vi "LDA_Angle_Checks.vi"(0 "Vg1":dbl[](array[numeric])=[-0.9913846154927373, -0.08722653267640797, -0.09771425771896834] format="%#.3g", 1 "Vg2":dbl[](array[numeric])=[-0.987756229722306, 0.06610682889995216, -0.1413064677131501] format="%#.3g", 2 "Vb1":dbl[](array[numeric])=[-0.9989930425665134, 0.011295311772511737, -0.04342023532481111] format="%#.3g", 3 "Vb2":dbl[](array[numeric])=[-0.9801478026485297, -0.032415015548967537, -0.19560049010730732] format="%#.3g") -> (6 "Vp from Greens":dbl[](array[numeric])=[-0.9927304194336236, -0.01059357268028935, -0.11989199535001964] format="%.3f", 7 "Vp from Blues":dbl[](array[numeric])=[-0.9927304194336236, -0.010593572680289348, -0.11989199535001965] format="%.3f", 8 "Angle between beam planes (deg)":dbl=90.0 format="%#.3g", 9 "Vp difference (G-B)":dbl[](array[numeric])=[0.0, -1.734723475976807e-18, 1.3877787807814457e-17] format="%_3f", 10 "Angle of spot B1 corner (deg)":dbl=89.99999914622636 format="%#.3g", 11 "Angle of spot B2 corner (deg)":dbl=90.0 format="%#.3g", 12 "Angle of spot G1 corner (deg)":dbl=90.0 format="%#.3g", 13 "Angle of spot G2 corner (deg)":dbl=89.99999914622636 format="%#.3g", 14 "Green divergence angle (deg)":dbl=9.14556525944418 format="%#.3g", 15 "Blue divergence angle (deg)":dbl=9.14556525944422 format="%#.3g", 16 "Angle between Vg1 and Vb1 (deg)":dbl=6.4634547293452185 format="%#.3g", 17 "Angle between Vg1 and Vb2 (deg)":dbl=6.4634547293452185 format="%#.3g", 18 "Angle between Vg2 and Vb1 (deg)":dbl=6.463454729345162 format="%#.3g", 19 "Angle between Vg2 and Vb2 (deg)":dbl=6.463454729345162 format="%#.3g")   [LabVIEW 2010]
uses:
  <vilib>/Analysis/baseanly.llb/Unit Vector (DBL).vi
  <vilib>/Analysis/baseanly.llb/Real Dot Product.vi
  <vilib>/Analysis/NI_AALBase.lvlib
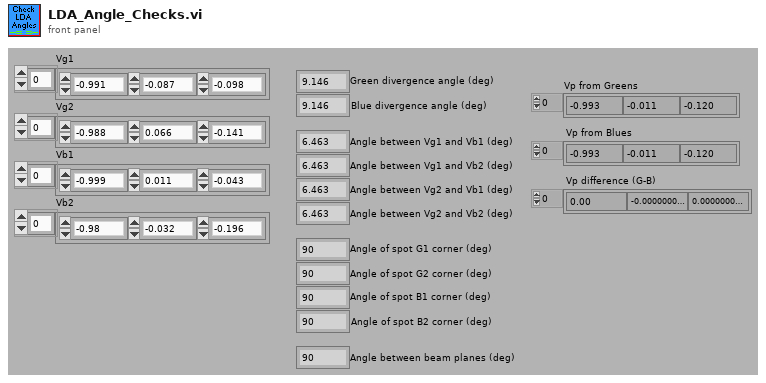
[diagram p1: front panel]
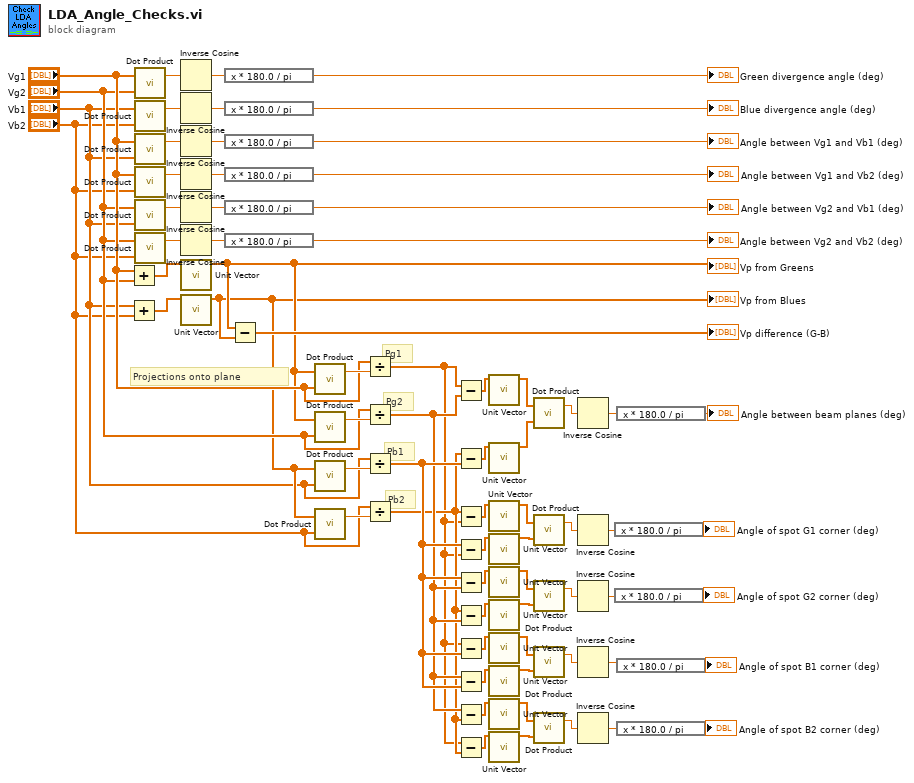
[diagram p0: block diagram]
diagram:
  # "Pb2"
  # "Pb1"
  # "Pg2"
  # "Pg1"
  # "Projections onto plane"
  n1 = Add(x="Vg1", y="Vg2") -> (x+y=w52:dbl[])
  n2 = Add(x="Vb1", y="Vb2") -> (x+y=w51:dbl[])
  n3 = call-poly <vilib>:"Dot Product.vi"("Y Vector"="Vg2", "X Vector"="Vg1") -> ("X * Y"=w64:dbl)  [unwired: 1 out]
  n4 = call-poly <vilib>:"Dot Product.vi"("Y Vector"="Vb2", "X Vector"="Vb1") -> ("X * Y"=w63:dbl)  [unwired: 1 out]
  n5 = call-poly <vilib>:"Dot Product.vi"("Y Vector"="Vb1", "X Vector"="Vg1") -> ("X * Y"=w62:dbl)  [unwired: 1 out]
  n6 = call-poly <vilib>:"Dot Product.vi"("Y Vector"="Vb2", "X Vector"="Vg1") -> ("X * Y"=w61:dbl)  [unwired: 1 out]
  n7 = call-poly <vilib>:"Dot Product.vi"("Y Vector"="Vb1", "X Vector"="Vg2") -> ("X * Y"=w60:dbl)  [unwired: 1 out]
  n8 = call-poly <vilib>:"Dot Product.vi"("Y Vector"="Vb2", "X Vector"="Vg2") -> ("X * Y"=w59:dbl)  [unwired: 1 out]
  n9 = Inverse Cosine(1:w64) -> (0:w69:dbl)
  n10 = Inverse Cosine(1:w63) -> (0:w70:dbl)
  n11 = Inverse Cosine(1:w62) -> (0:w68:dbl)
  n12 = Inverse Cosine(1:w61) -> (0:w67:dbl)
  n13 = Inverse Cosine(1:w60) -> (0:w66:dbl)
  n14 = Inverse Cosine(1:w59) -> (0:w65:dbl)
  n15 = call-poly <vilib>:"Unit Vector.vi"("Input Vector"=w52) -> ("Unit Vector"=w45:dbl[])  [unwired: 2 in, 8 out]
  "Vp from Greens" <- w45
  n16 = call-poly <vilib>:"Unit Vector.vi"("Input Vector"=w51) -> ("Unit Vector"=w42:dbl[])  [unwired: 2 in, 8 out]
  "Vp from Blues" <- w42
  n17 = expression code="x * 180.0 / pi"(w69) -> (→"Green divergence angle (deg)":dbl)
  n18 = expression code="x * 180.0 / pi"(w70) -> (→"Blue divergence angle (deg)":dbl)
  n19 = expression code="x * 180.0 / pi"(w68) -> (→"Angle between Vg1 and Vb1 (deg)":dbl)
  n20 = expression code="x * 180.0 / pi"(w67) -> (→"Angle between Vg1 and Vb2 (deg)":dbl)
  n21 = expression code="x * 180.0 / pi"(w66) -> (→"Angle between Vg2 and Vb1 (deg)":dbl)
  n22 = expression code="x * 180.0 / pi"(w65) -> (→"Angle between Vg2 and Vb2 (deg)":dbl)
  n23 = Subtract(x=w45, y=w42) -> (x-y=→"Vp difference (G-B)":dbl[])
  n24 = call-poly <vilib>:"Dot Product.vi"("Y Vector"="Vg1", "X Vector"=w45) -> ("X * Y"=w49:dbl)  [unwired: 1 out]
  n25 = call-poly <vilib>:"Dot Product.vi"("Y Vector"="Vg2", "X Vector"=w45) -> ("X * Y"=w47:dbl)  [unwired: 1 out]
  n26 = call-poly <vilib>:"Dot Product.vi"("Y Vector"="Vb1", "X Vector"=w42) -> ("X * Y"=w43:dbl)  [unwired: 1 out]
  n27 = call-poly <vilib>:"Dot Product.vi"("Y Vector"="Vb2", "X Vector"=w42) -> ("X * Y"=w44:dbl)  [unwired: 1 out]
  n28 = Divide(x="Vg1", y=w49) -> (x/y=w21:dbl[])
  n29 = Divide(x="Vg2", y=w47) -> (x/y=w23:dbl[])
  n30 = Divide(x="Vb1", y=w43) -> (x/y=w24:dbl[])
  n31 = Divide(x="Vb2", y=w44) -> (x/y=w22:dbl[])
  n32 = Subtract(x=w21, y=w23) -> (x-y=w38:dbl[])
  n33 = Subtract(x=w22, y=w24) -> (x-y=w39:dbl[])
  n34 = Subtract(x=w22, y=w21) -> (x-y=w36:dbl[])
  n35 = Subtract(x=w24, y=w21) -> (x-y=w35:dbl[])
  n36 = Subtract(x=w24, y=w23) -> (x-y=w31:dbl[])
  n37 = Subtract(x=w22, y=w23) -> (x-y=w32:dbl[])
  n38 = Subtract(x=w21, y=w24) -> (x-y=w25:dbl[])
  n39 = Subtract(x=w23, y=w24) -> (x-y=w26:dbl[])
  n40 = Subtract(x=w23, y=w22) -> (x-y=w30:dbl[])
  n41 = Subtract(x=w21, y=w22) -> (x-y=w29:dbl[])
  n42 = call-poly <vilib>:"Unit Vector.vi"("Input Vector"=w38) -> ("Unit Vector"=w20:dbl[])  [unwired: 2 in, 8 out]
  n43 = call-poly <vilib>:"Unit Vector.vi"("Input Vector"=w39) -> ("Unit Vector"=w19:dbl[])  [unwired: 2 in, 8 out]
  n44 = call-poly <vilib>:"Unit Vector.vi"("Input Vector"=w36) -> ("Unit Vector"=w7:dbl[])  [unwired: 2 in, 8 out]
  n45 = call-poly <vilib>:"Unit Vector.vi"("Input Vector"=w35) -> ("Unit Vector"=w6:dbl[])  [unwired: 2 in, 8 out]
  n46 = call-poly <vilib>:"Unit Vector.vi"("Input Vector"=w31) -> ("Unit Vector"=w5:dbl[])  [unwired: 2 in, 8 out]
  n47 = call-poly <vilib>:"Unit Vector.vi"("Input Vector"=w32) -> ("Unit Vector"=w4:dbl[])  [unwired: 2 in, 8 out]
  n48 = call-poly <vilib>:"Unit Vector.vi"("Input Vector"=w25) -> ("Unit Vector"=w11:dbl[])  [unwired: 2 in, 8 out]
  n49 = call-poly <vilib>:"Unit Vector.vi"("Input Vector"=w26) -> ("Unit Vector"=w10:dbl[])  [unwired: 2 in, 8 out]
  n50 = call-poly <vilib>:"Unit Vector.vi"("Input Vector"=w30) -> ("Unit Vector"=w12:dbl[])  [unwired: 2 in, 8 out]
  n51 = call-poly <vilib>:"Unit Vector.vi"("Input Vector"=w29) -> ("Unit Vector"=w1:dbl[])  [unwired: 2 in, 8 out]
  n52 = call-poly <vilib>:"Dot Product.vi"("Y Vector"=w19, "X Vector"=w20) -> ("X * Y"=w18:dbl)  [unwired: 1 out]
  n53 = call-poly <vilib>:"Dot Product.vi"("Y Vector"=w6, "X Vector"=w7) -> ("X * Y"=w16:dbl)  [unwired: 1 out]
  n54 = call-poly <vilib>:"Dot Product.vi"("Y Vector"=w4, "X Vector"=w5) -> ("X * Y"=w15:dbl)  [unwired: 1 out]
  n55 = call-poly <vilib>:"Dot Product.vi"("Y Vector"=w10, "X Vector"=w11) -> ("X * Y"=w14:dbl)  [unwired: 1 out]
  n56 = call-poly <vilib>:"Dot Product.vi"("Y Vector"=w1, "X Vector"=w12) -> ("X * Y"=w13:dbl)  [unwired: 1 out]
  n57 = Inverse Cosine(1:w18) -> (0:w17:dbl)
  n58 = Inverse Cosine(1:w16) -> (0:w3:dbl)
  n59 = Inverse Cosine(1:w15) -> (0:w2:dbl)
  n60 = Inverse Cosine(1:w14) -> (0:w9:dbl)
  n61 = Inverse Cosine(1:w13) -> (0:w8:dbl)
  n62 = expression code="x * 180.0 / pi"(w3) -> (→"Angle of spot G1 corner (deg)":dbl)
  n63 = expression code="x * 180.0 / pi"(w2) -> (→"Angle of spot G2 corner (deg)":dbl)
  n64 = expression code="x * 180.0 / pi"(w17) -> (→"Angle between beam planes (deg)":dbl)
  n65 = expression code="x * 180.0 / pi"(w9) -> (→"Angle of spot B1 corner (deg)":dbl)
  n66 = expression code="x * 180.0 / pi"(w8) -> (→"Angle of spot B2 corner (deg)":dbl)
